vi "cornell-Ktildesh2sides.vi"(0 "ω":cdb=10.0+0.0i, 1 "s":dbl=0.5, 2 "τGright":dbl=1.0, 3 "h":dbl=0.5, 4 "τGleft":dbl=1.0, 5 "τS":dbl=1.0, 7 "#of terms":i64=500, 8 "action":T1) -> (19 "Ks(ω)":cdb=1.1764208086940058-0.8519213260397617i)   [LabVIEW 2020]
uses:
  cornell-Ktildesh2sides.ctl
  cornell-K0s.vi
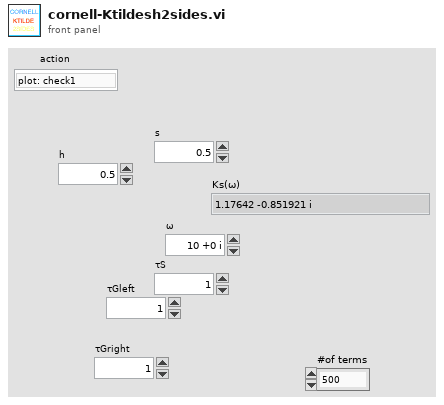
[diagram p1: front panel]
types:
  T1 = typedef "cornell-Ktildesh2sides.ctl" = enum16{"plot: check1", "plot: check2", "plot: one½", "plot: two½", "plot: uni½", "calc: zcoth(z)", "calc: z/sinh(z)", "calc: brute", "calc: integra", "void"}
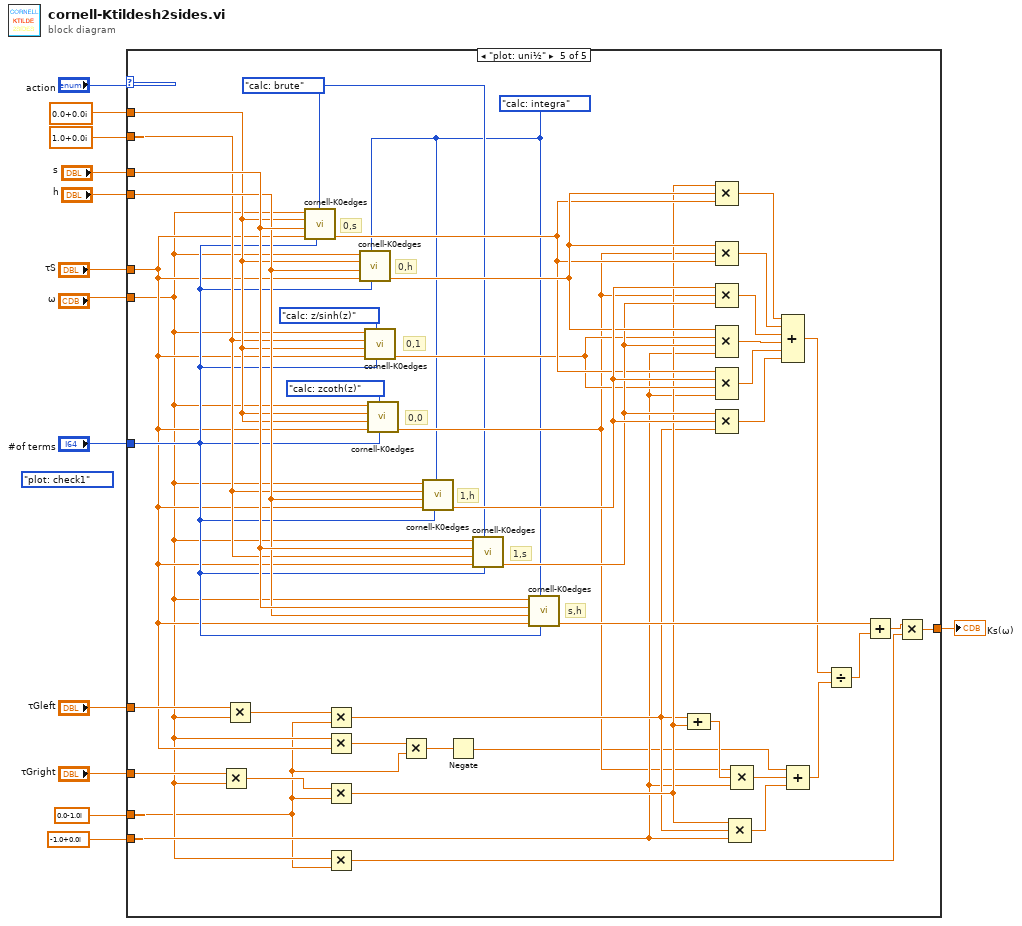
[diagram p0: block diagram]
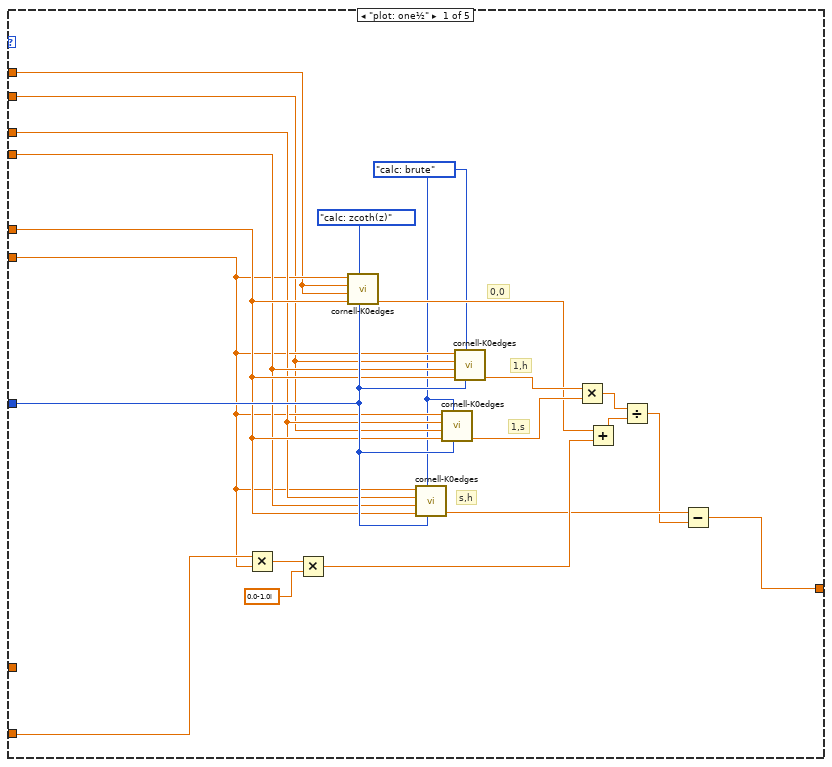
[diagram p2: hidden frame]
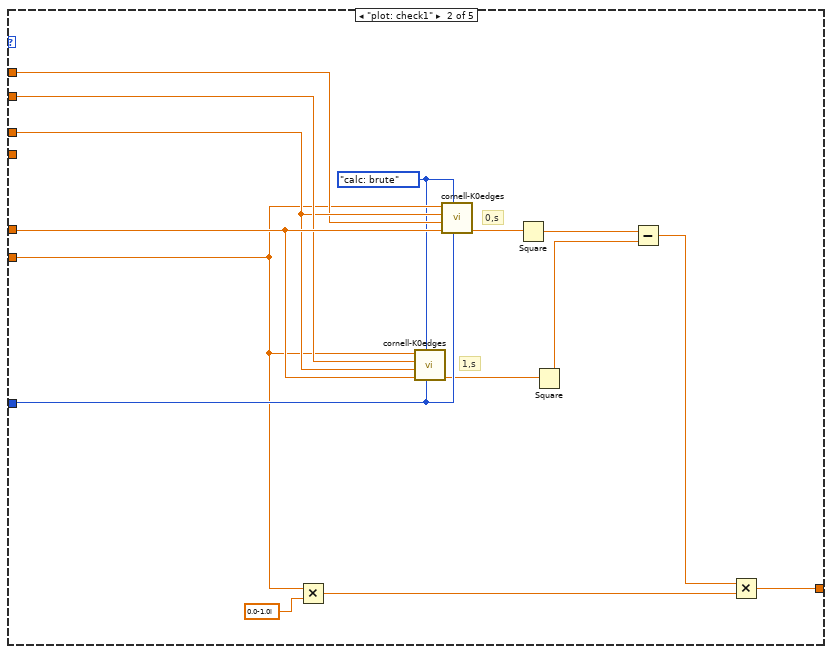
[diagram p3: hidden frame]
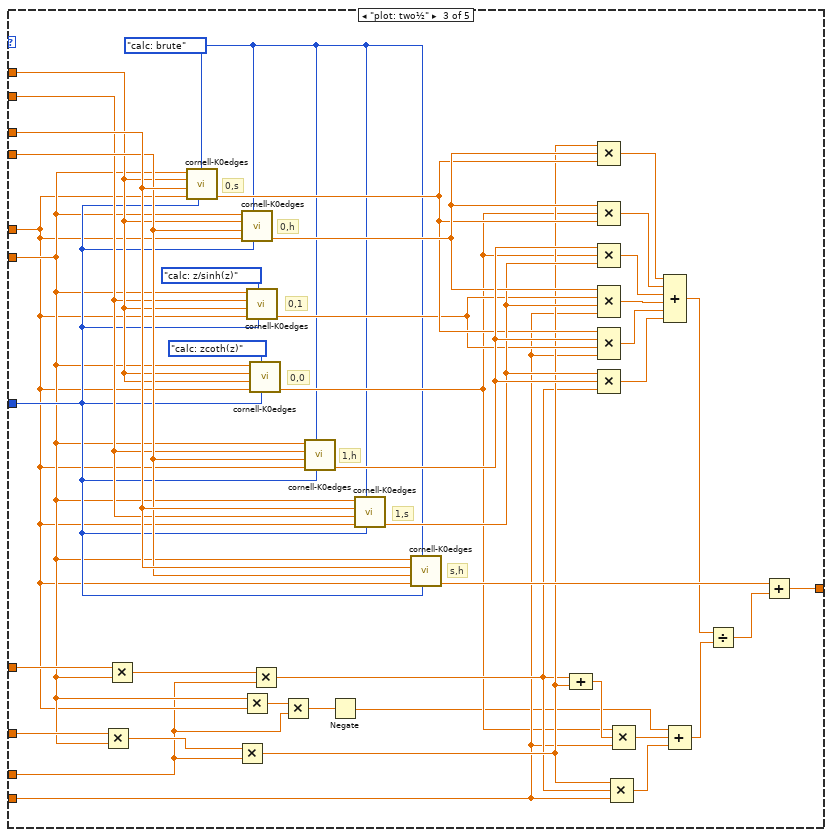
[diagram p4: hidden frame]
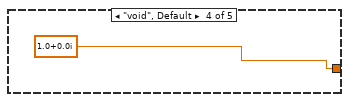
[diagram p5: hidden frame]
diagram:
  (unwired) cornell-Ktildesh2sides."plot: check1"
  n1 = case shown="\"plot: uni½\"" "action" {
    tunnel: "τGleft" -> [_ _ w89 _ w134]
    tunnel: [w24 w44 w88 cdb 1.0+0.0i ("s") w92] -> w12
    tunnel: "τGright" -> [w23 _ w84 _ w130]
    tunnel: "s" -> [w19 w42 w83 _ w129]
    tunnel: "h" -> [w20 _ w82 _ w128]
    tunnel: "ω" -> [w18 w36 w57 _ w96]
    tunnel: "τS" -> [w21 w47 w56 _ w103]
    tunnel: cdb 0.0+0.0i ("h") -> [w16 w41 w81 _ w127]
    tunnel: cdb 1.0+0.0i ("s") -> [w17 w43 w80 _ w126]
    tunnel: cdb -1.0+0.0i ("s") -> [_ _ w65 _ w111]
    tunnel: "#of terms" -> [w22 w48 w60 _ w106]
    tunnel: cdb 0.0-1.0i ("x") -> [_ _ w55 _ w95]
    frame "plot: one½" {
      w14 = cornell-Ktildesh2sides."calc: brute" ("secelt")
      # "0,0"
      # "1,s"
      # "1,h"
      # "s,h"
      n2 = Multiply(x=w23, y=w18) -> (x*y=w34:cdb)
      n3 = Multiply(x=w34, y=cdb 0.0-1.0i ("x")) -> (x*y=w30:cdb)
      n4 = call "cornell-K0edges.vi"("Numeric"=w22, "secelt"=cornell-Ktildesh2sides."calc: zcoth(z)", "τ"=w21, "h"=w16, "s"=w16, "ω"=w18) -> ("Ks(ω)"=w29:cdb)  [unwired: 5 in]
      n5 = call "cornell-K0edges.vi"("Numeric"=w22, "secelt"=w14, "τ"=w21, "h"=w20, "s"=w19, "ω"=w18) -> ("Ks(ω)"=w26:cdb)  [unwired: 5 in]
      n6 = call "cornell-K0edges.vi"("Numeric"=w22, "secelt"=w14, "τ"=w21, "h"=w17, "s"=w19, "ω"=w18) -> ("Ks(ω)"=w31:cdb)  [unwired: 5 in]
      n7 = call "cornell-K0edges.vi"("Numeric"=w22, "secelt"=w14, "τ"=w21, "h"=w20, "s"=w17, "ω"=w18) -> ("Ks(ω)"=w32:cdb)  [unwired: 5 in]
      n8 = Multiply(x=w32, y=w31) -> (x*y=w28:cdb)
      n9 = Add(x=w29, y=w30) -> (x+y=w27:cdb)
      n10 = Divide(x=w28, y=w27) -> (x/y=w25:cdb)
      n11 = Subtract(x=w26, y=w25) -> (x-y=w24:cdb)
    }
    frame "plot: check1" {
      w35 = cornell-Ktildesh2sides."calc: brute" ("secelt")
      # "0,s"
      # "1,s"
      n12 = Multiply(x=w36, y=cdb 0.0-1.0i ("x")) -> (x*y=w45:cdb)
      n13 = call "cornell-K0edges.vi"("Numeric"=w48, "secelt"=w35, "τ"=w47, "h"=w42, "s"=w43, "ω"=w36) -> ("Ks(ω)"=w40:cdb)  [unwired: 5 in]
      n14 = call "cornell-K0edges.vi"("Numeric"=w48, "secelt"=w35, "τ"=w47, "h"=w41, "s"=w42, "ω"=w36) -> ("Ks(ω)"=w39:cdb)  [unwired: 5 in]
      n15 = Square(x=w39) -> (x^2=w37:cdb)
      n16 = Square(x=w40) -> (x^2=w38:cdb)
      n17 = Subtract(x=w37, y=w38) -> (x-y=w46:cdb)
      n18 = Multiply(x=w46, y=w45) -> (x*y=w44:cdb)
    }
    frame "plot: two½" {
      w50 = cornell-Ktildesh2sides."calc: brute" ("secelt")
      # "0,s"
      # "0,h"
      # "0,1"
      # "0,0"
      # "1,s"
      # "1,h"
      # "s,h"
      n19 = Multiply(x=w84, y=w57) -> (x*y=w85:cdb)
      n20 = Multiply(x=w89, y=w57) -> (x*y=w90:cdb)
      n21 = call "cornell-K0edges.vi"("Numeric"=w60, "secelt"=w50, "τ"=w56, "h"=w83, "s"=w81, "ω"=w57) -> ("Ks(ω)"=w76:cdb)  [unwired: 5 in]
      n22 = Multiply(x=w85, y=w55) -> (x*y=w67:cdb)
      n23 = call "cornell-K0edges.vi"("Numeric"=w60, "secelt"=w50, "τ"=w56, "h"=w82, "s"=w81, "ω"=w57) -> ("Ks(ω)"=w78:cdb)  [unwired: 5 in]
      n24 = Multiply(x=w57, y=w56) -> (x*y=w58:cdb)
      n25 = call "cornell-K0edges.vi"("Numeric"=w60, "secelt"=cornell-Ktildesh2sides."calc: z/sinh(z)", "τ"=w56, "h"=w81, "s"=w80, "ω"=w57) -> ("Ks(ω)"=w69:cdb)  [unwired: 5 in]
      n26 = call "cornell-K0edges.vi"("Numeric"=w60, "secelt"=cornell-Ktildesh2sides."calc: zcoth(z)", "τ"=w56, "h"=w81, "s"=w81, "ω"=w57) -> ("Ks(ω)"=w59:cdb)  [unwired: 5 in]
      n27 = Multiply(x=w90, y=w55) -> (x*y=w66:cdb)
      n28 = Multiply(x=w58, y=w55) -> (x*y=w54:cdb)
      n29 = call "cornell-K0edges.vi"("Numeric"=w60, "secelt"=w50, "τ"=w56, "h"=w82, "s"=w80, "ω"=w57) -> ("Ks(ω)"=w79:cdb)  [unwired: 5 in]
      n30 = Negate(x=w54) -> (-x=w53:cdb)
      n31 = call "cornell-K0edges.vi"("Numeric"=w60, "secelt"=w50, "τ"=w56, "h"=w80, "s"=w83, "ω"=w57) -> ("Ks(ω)"=w77:cdb)  [unwired: 5 in]
      n32 = call "cornell-K0edges.vi"("Numeric"=w60, "secelt"=w50, "τ"=w56, "h"=w82, "s"=w83, "ω"=w57) -> ("Ks(ω)"=w87:cdb)  [unwired: 5 in]
      n33 = Compound Arithmetic op=ADD(w66, w67) -> (w68:cdb)
      n34 = Compound Arithmetic op=MULTIPLY(w67, w78, w76) -> (w75:cdb)
      n35 = Compound Arithmetic op=MULTIPLY(w78, w59, w76) -> (w74:cdb)
      n36 = Compound Arithmetic op=MULTIPLY(w79, w59, w77) -> (w73:cdb)
      n37 = Compound Arithmetic op=MULTIPLY(w78, w69, w77, w65) -> (w72:cdb)
      n38 = Compound Arithmetic op=MULTIPLY(w76, w79, w69, w65) -> (w71:cdb)
      n39 = Compound Arithmetic op=MULTIPLY(w77, w79, w66) -> (w70:cdb)
      n40 = Compound Arithmetic op=MULTIPLY(w67, w66, w65) -> (w63:cdb)
      n41 = Compound Arithmetic op=MULTIPLY(w59, w68, w65) -> (w64:cdb)
      n42 = Compound Arithmetic op=ADD(w75, w74, w73, w72, w71, w70) -> (w62:cdb)
      n43 = Compound Arithmetic op=ADD(w53, w64, w63) -> (w61:cdb)
      n44 = Divide(x=w62, y=w61) -> (x/y=w86:cdb)
      n45 = Add(x=w87, y=w86) -> (x+y=w88:cdb)
    }
    frame "void", Default {
    }
    frame "plot: uni½" {
      w97 = cornell-Ktildesh2sides."calc: integra" ("secelt")
      w98 = cornell-Ktildesh2sides."calc: brute" ("secelt")
      # "0,s"
      # "0,h"
      # "0,1"
      # "0,0"
      # "1,s"
      # "1,h"
      # "s,h"
      n46 = Multiply(x=w130, y=w96) -> (x*y=w131:cdb)
      n47 = Multiply(x=w134, y=w96) -> (x*y=w135:cdb)
      n48 = call "cornell-K0edges.vi"("Numeric"=w106, "secelt"=w98, "τ"=w103, "h"=w129, "s"=w127, "ω"=w96) -> ("Ks(ω)"=w122:cdb)  [unwired: 5 in]
      n49 = Multiply(x=w135, y=w95) -> (x*y=w112:cdb)
      n50 = Multiply(x=w96, y=w103) -> (x*y=w104:cdb)
      n51 = Multiply(x=w131, y=w95) -> (x*y=w113:cdb)
      n52 = Multiply(x=w96, y=w95) -> (x*y=w93:cdb)
      n53 = call "cornell-K0edges.vi"("Numeric"=w106, "secelt"=w97, "τ"=w103, "h"=w128, "s"=w127, "ω"=w96) -> ("Ks(ω)"=w124:cdb)  [unwired: 5 in]
      n54 = call "cornell-K0edges.vi"("Numeric"=w106, "secelt"=cornell-Ktildesh2sides."calc: z/sinh(z)", "τ"=w103, "h"=w127, "s"=w126, "ω"=w96) -> ("Ks(ω)"=w115:cdb)  [unwired: 5 in]
      n55 = call "cornell-K0edges.vi"("Numeric"=w106, "secelt"=cornell-Ktildesh2sides."calc: zcoth(z)", "τ"=w103, "h"=w127, "s"=w127, "ω"=w96) -> ("Ks(ω)"=w105:cdb)  [unwired: 5 in]
      n56 = Multiply(x=w104, y=w95) -> (x*y=w102:cdb)
      n57 = call "cornell-K0edges.vi"("Numeric"=w106, "secelt"=w97, "τ"=w103, "h"=w128, "s"=w126, "ω"=w96) -> ("Ks(ω)"=w125:cdb)  [unwired: 5 in]
      n58 = Negate(x=w102) -> (-x=w101:cdb)
      n59 = call "cornell-K0edges.vi"("Numeric"=w106, "secelt"=w98, "τ"=w103, "h"=w126, "s"=w129, "ω"=w96) -> ("Ks(ω)"=w123:cdb)  [unwired: 5 in]
      n60 = call "cornell-K0edges.vi"("Numeric"=w106, "secelt"=w97, "τ"=w103, "h"=w128, "s"=w129, "ω"=w96) -> ("Ks(ω)"=w133:cdb)  [unwired: 5 in]
      n61 = Compound Arithmetic op=ADD(w112, w113) -> (w114:cdb)
      n62 = Compound Arithmetic op=MULTIPLY(w113, w124, w122) -> (w121:cdb)
      n63 = Compound Arithmetic op=MULTIPLY(w124, w105, w122) -> (w120:cdb)
      n64 = Compound Arithmetic op=MULTIPLY(w125, w105, w123) -> (w119:cdb)
      n65 = Compound Arithmetic op=MULTIPLY(w124, w115, w123, w111) -> (w118:cdb)
      n66 = Compound Arithmetic op=MULTIPLY(w122, w125, w115, w111) -> (w117:cdb)
      n67 = Compound Arithmetic op=MULTIPLY(w123, w125, w112) -> (w116:cdb)
      n68 = Compound Arithmetic op=MULTIPLY(w113, w112, w111) -> (w109:cdb)
      n69 = Compound Arithmetic op=MULTIPLY(w105, w114, w111) -> (w110:cdb)
      n70 = Compound Arithmetic op=ADD(w121, w120, w119, w118, w117, w116) -> (w108:cdb)
      n71 = Compound Arithmetic op=ADD(w101, w110, w109) -> (w107:cdb)
      n72 = Divide(x=w108, y=w107) -> (x/y=w132:cdb)
      n73 = Add(x=w133, y=w132) -> (x+y=w94:cdb)
      n74 = Multiply(x=w94, y=w93) -> (x*y=w92:cdb)
    }
  }
  "Ks(ω)" <- w12
